vi "DefaultFromINI.vi"(8 "error in (no error)":errorcluster, 11 "NHRDCModel":refnum<class "NHRDCPowerModel.lvclass">) -> (0 "error out":errorcluster, 3 "NHRDCModel":refnum<class "NHRDCPowerModel.lvclass">)   [LabVIEW 2018, in "AcPwrPlugins.lvlib" / "NHRDCPowerModel.lvclass"]
doc: "This VI loads the instruments' configuration previously stored on file."
uses:
  NHRDCPowerModel.lvclass
  F:/Program Files (x86)/National Instruments/LabVIEW 2018/user.lib/NIST/BaseClasses/BasePlugin_class/BasePlugin.lvclass
  F:/Projects/ICDAS/NistPluggableModules/AcPwr/AcPwrPlugins/AcPwrBaseClass/AcPwrBase.lvclass
  NHRDCPowerClass/TypeDefs/Device(s)Settings.ctl
  NHRDCPowerClass/TypeDefs/Modules.ctl
  NHRDCPowerClass/TypeDefs/Measurements.ctl
  AcPwrShared/Database Settings.ctl
  <userlib>/NIST/BaseClasses/BasePlugin_class/BasePlugin.lvclass/BasePlugin.ctl
  <userlib>/NIST/BaseClasses/BasePlugin_class/Accessors/Read PluginIniFilePath.vi
  AcPwrBaseClass/AcPwrBase.lvclass
  <vilib>/Utility/config.llb/NI_LVConfig.lvlib
  NHRDCPowerClass/NHRDCPower.lvclass
  AcPwrShared/AcPwrShared.lvlib
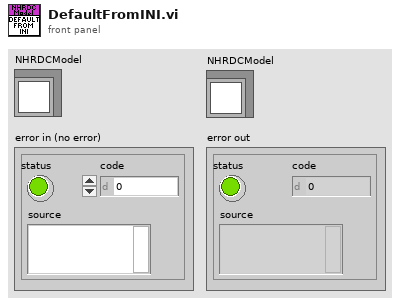
[diagram p1: front panel]
types:
  T1 = typedef "AcPwrShared.lvlib/Database Settings.ctl" = cluster{"Data Source":string, "ICDAS to Model Table":string, "Model to ICDAS Table":string}
  T2 = typedef "AcPwrPlugins.lvlib/NHRDCPower.lvclass/Measurements.ctl" = cluster{"Handle":string, "Name":string, "Enabled":bool, "Measurement Value":sgl, "Measurement Type":enum16{"Power", "Current", "Voltage"}}[]
  T3 = typedef "AcPwrPlugins.lvlib/NHRDCPower.lvclass/Device(s)Settings.ctl" = cluster{"MeasName":string, "Modules":T4}
  T4 = typedef "AcPwrPlugins.lvlib/NHRDCPower.lvclass/Modules.ctl" = cluster{"Handle":string, "Name":string, "id query (Yes)":bool, "reset device (Yes)":bool, "Connected":bool, "Initial Battery Detect Voltage (0)":dbl, "SafetySettings":cluster{"SetWatchDog?":bool, "Voltage (V)":dbl, "Current (A)":dbl, "Power (W)":dbl, "Voltage Delay (s)":dbl, "Current Delay (s)":dbl, "Power Delay (s)":dbl}, "Options String":string, "Aperture Time (s)":dbl, "operating state (Off)":i32, "OutputSettings":cluster{"Voltage (V)":dbl, "Current (A)":dbl, "Resistance (Ohms)":dbl, "Power (W)":dbl, "Enable Voltage":bool, "Enable Current":bool, "Enable Resistance":bool, "Enable Power":bool, "Macro After Step Delay  (s)":dbl, "Wait Value (V, A, W)":dbl, "Enable Wait":bool, "Wait on Value":i32}, "SlewRate":cluster{"Set Voltage Rate V/S":dbl, "Set Current Rate A/S":dbl, "Set Resistance Rate R/S":dbl, "Set Power Rate W/S":dbl}, "Macro":cluster{"Save Macro?":bool, "Load Macro From File?":bool, "Run Macro Continuously?":bool, "Use Macros?":bool, "Load Macro File Path":path, "Save Macro File Path":string}, "Regulation Gain (1=100%)":dbl, "UpdatingOntheFly":bool}[]
  T5 = typedef "NI_LVConfig.lvlib/Config Data RefNum.ctl" = refnum<k1>
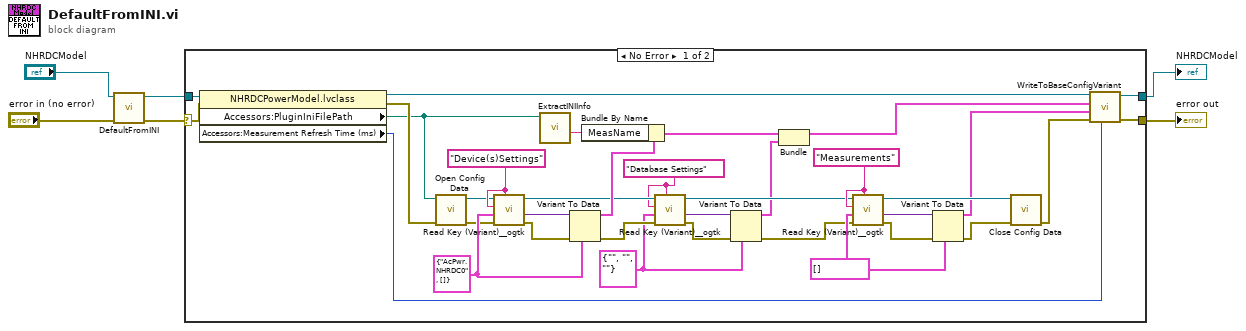
[diagram p0: block diagram]
diagram:
  n1 = call-parent "DefaultFromINI.vi"("error in (no error)"="error in (no error)", "AcPwrBase"="NHRDCModel") -> ("error out"=w4:errorcluster, "AcPwrBase"=w3:refnum<class "NHRDCPowerModel.lvclass">)  [unwired: 8 in]
  n2 = case shown="No Error" w4 {
    selector: w4 -> [w40 w42]
    tunnel: [w38 w43] -> w2
    tunnel: w3 -> [w41 w43]
    tunnel: [w39 w42] -> w1
    frame No Error {
      w14 = T1 {"Data Source"="", "ICDAS to Model Table"="", "Model to ICDAS Table"=""} ("Database Settings")
      w16 = "Database Settings" ("section")
      w28 = T2 [] ("Measurements")
      w29 = "Measurements" ("section")
      w34 = "Device(s)Settings" ("section")
      w35 = T3 {"MeasName"="AcPwr.NHRDC0", "Modules"=[]} ("NHRDC")
      n3 = property class="NHRDCPowerModel.lvclass"(reference=w41, error in=w40) -> (reference out=w36:refnum<class "NHRDCPowerModel.lvclass">, error out=w37:errorcluster, "Accessors:PluginIniFilePath"=w20:path, "Accessors:Measurement Refresh Time (ms)"=w22:u32)
      n4 = call <vilib>:"Open Config Data.vi"("error in (no error)"=w37, "configuration file path"=w20) -> ("error out"=w32:errorcluster, "refnum"=w33:T5)  [unwired: 7 in, 1 out]
      n5 = call <userlib>:"Read Key (Variant)__ogtk.vi"("section"=w34, "error in (no error)"=w32, "type"=w35, "key (optional)"=w34, "refnum"=w33) -> ("error out"=w31:errorcluster, "key-value"=w30:variant, "refnum out"=w18:T5)  [unwired: 3 in, 1 out]
      n6 = call "ExtractINIInfo.vi"("INI File Path"=w20) -> ("Plugin Name"=w19:string)  [unwired: 8 in, 2 out]
      n7 = Variant To Data(error in=w31, type=w35, Variant=w30) -> (data=w21:T3, error out=w17:errorcluster)
      n8 = Bundle By Name(cluster=w21, "MeasName"=w19) -> (w9:T3)
      n9 = call <userlib>:"Read Key (Variant)__ogtk.vi"("section"=w16, "error in (no error)"=w17, "type"=w14, "key (optional)"=w16, "refnum"=w18) -> ("error out"=w15:errorcluster, "key-value"=w13:variant, "refnum out"=w12:T5)  [unwired: 3 in, 1 out]
      n10 = Variant To Data(error in=w15, type=w14, Variant=w13) -> (data=w8:T1, error out=w11:errorcluster)
      n11 = Bundle("NHRDC"=w9, "Database Settings"=w8) -> (w10:cluster{"NHRDC":T3, "Database Settings":T1})  [unwired: 1 in]
      n12 = call <userlib>:"Read Key (Variant)__ogtk.vi"("section"=w29, "error in (no error)"=w11, "type"=w28, "key (optional)"=w29, "refnum"=w12) -> ("error out"=w27:errorcluster, "key-value"=w26:variant, "refnum out"=w25:T5)  [unwired: 3 in, 1 out]
      n13 = Variant To Data(error in=w27, type=w28, Variant=w26) -> (data=w23:T2, error out=w24:errorcluster)
      n14 = call <vilib>:"Close Config Data.vi"("error in (no error)"=w24, "refnum"=w25) -> ("error out"=w7:errorcluster)  [unwired: 8 in, 1 out]
      n15 = call-dynamic "WriteToBaseConfigVariant.vi"("Measurement Refresh Time (ms)"=w22, "error in (no error)"=w7, "Meas"=w23, "Config"=w10, "NHRDCModel in"=w36) -> ("error out"=w39:errorcluster, "NHRDCModel out"=w38:refnum<class "NHRDCPowerModel.lvclass">)  [unwired: 5 in]
    }
    frame Error {
    }
  }
  "error out" <- w1
  "NHRDCModel" <- w2
